vi "NextGUIState.vi"(8 "Error In":errorcluster, 9 "State Argument":string, 10 "GUI State":string, 11 "Queue In":refnum<queue>) -> (0 "Error Out":errorcluster, 3 "Queue Out":refnum<queue>)   [LabVIEW 2010]
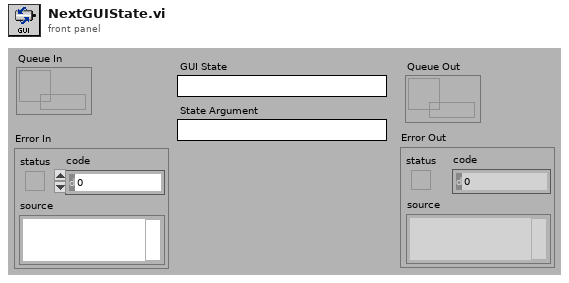
[diagram p1: front panel]
types:
  T1 = cluster{"GUI State":string, "State Argument":string}
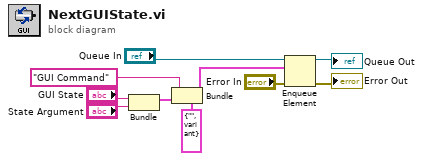
[diagram p0: block diagram]
diagram:
  n1 = Bundle("GUI State"="GUI State", "State Argument"="State Argument") -> (w3:T1)  [unwired: 1 in]
  n2 = Bundle(cluster=cluster{"State":string, "Data":variant} {"State"="", "Data"=variant} ("output cluster"), "State"="GUI Command", "Data"=w3) -> (w1:cluster{"State":string, "Data":variant})
  n3 = Enqueue Element(queue="Queue In", element=w1, error in (no error)="Error In") -> (queue out=→"Queue Out":refnum<queue>, error out=→"Error Out":errorcluster)  [unwired: 1 in, 1 out]
